vi "UI.Addon.Path.Parse.vi"(11 "Cached Addon Path":string) -> (0 "Addon Name":string, 1 "IP Address":string, 2 "Controller and IP Address":string, 3 "Addon Path":string)   [LabVIEW 2019, in "Instrument Workspace Shared.lvlib"]
uses:
  Instrument Workspace Shared.lvlib
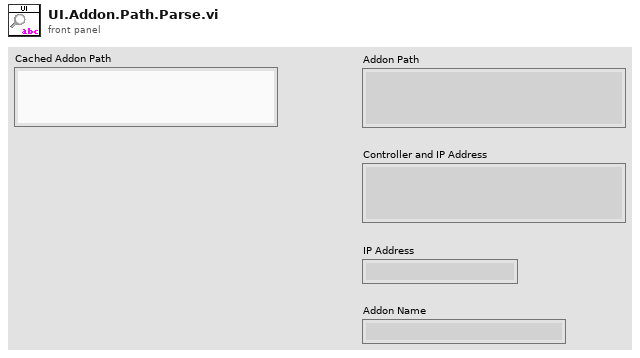
[diagram p1: front panel]
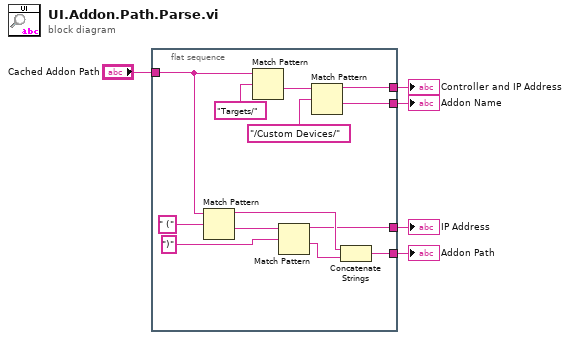
[diagram p0: block diagram]
diagram:
  n1 = flat-sequence {
    tunnel: [w12] -> w2
    tunnel: "Cached Addon Path" -> [w6]
    tunnel: [w14] -> w4
    tunnel: [w7] -> w5
    tunnel: [w11] -> w1
    frame #0 {
      n2 = Match Pattern(string=w6, regular expression=" (") -> (before substring=w15:string, after substring=w16:string)  [unwired: 1 in, 2 out]
      n3 = Match Pattern(string=w6, regular expression="Targets/") -> (after substring=w8:string)  [unwired: 1 in, 3 out]
      n4 = Match Pattern(string=w16, regular expression=")") -> (before substring=w12:string, after substring=w10:string)  [unwired: 1 in, 2 out]
      n5 = Match Pattern(string=w8, regular expression="/Custom Devices/") -> (before substring=w7:string, after substring=w11:string)  [unwired: 1 in, 2 out]
      n6 = Concatenate Strings(w15, w10) -> (w14:string)
    }
  }
  "Controller and IP Address" <- w5
  "Addon Path" <- w4
  "IP Address" <- w2
  "Addon Name" <- w1
